vi "FPGAcode4_Test2.vi"() -> ()   [LabVIEW 2015]
uses:
  Limits_In.ctl
  Detector_Cluster.ctl
  <vilib>/Platform/TimedLoop/XDataNode/timing_clust.ctl
  <vilib>/Platform/TimedLoop/XDataNode/nitl_modes.ctl
  <vilib>/Platform/TimedLoop/XDataNode/wakeup.ctl
  Correlations.ctl
  <vilib>/rvi/Emulation/niFpgaGetClockAttributes.vi
  <vilib>/rvi/Emulation/niFpgaSctlEmulationGetInTimedLoop.vi
  <vilib>/rvi/Emulation/niFpgaEmulationReportErrorSimple.vi
  <vilib>/rvi/Emulation/niFpgaProcessEmulError.vi
  <vilib>/rvi/eio/common/nirviEmuTemplateMethod_errors.vi
  <vilib>/rvi/Emulation/niFpgaCriticalErrorInLSC.vi
  <vilib>/eio/EIONode/EIONode.xnode
  <vilib>/Platform/TimedLoop/XDataNode/XDataNode.xnode
  <vilib>/Platform/TimedLoop/XDataNode/XDNodeRunTimeDep.lvlib
panel:
  out "Detectors":T1
  in  "User Trigger?":bool
  in  "User Trigger Distance":fxp<+/-,34,18> format="%.3g"
  out "User Trigger":bool
  in  "Charge Error Factor":fxp<+,32,0>=0.19999999995343387 format="%_2g"
  in  "Threshold Factor":fxp<+/-,32,16>=1.149993896484375 format="%.2g"
  out "DCS 2":bool
  out "DCS 1":bool
  in  "Limits":T2={"High Charge Limit"=4.54747350780585e-13, "Low Charge Limit"=0.0, "High Velocity Limit"=262143.0, "Low Velocity Limit"=0.0, "High Mass Limit"=7.27595761248936e-12, "Low Mass Limit"=0.0, "High Voltage"=2200000.0}
  in  "Calibrate":bool=TRUE
  in  "Armed":bool
  out "Plates":bool
  in  "One Shot":bool
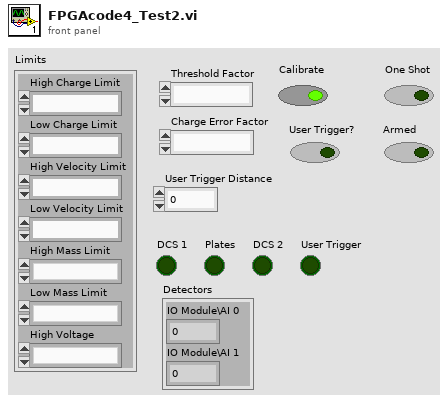
[diagram p1: front panel]
types:
  T1 = cluster{"IO Module\\AI 0":i16, "IO Module\\AI 1":i16}
  T2 = typedef "Limits_In.ctl" = cluster{"High Charge Limit":fxp<+,32,-41>, "Low Charge Limit":fxp<+,32,-41>, "High Velocity Limit":fxp<+,18,18>, "Low Velocity Limit":fxp<+,18,18>, "High Mass Limit":fxp<+/-,33,-36>, "Low Mass Limit":fxp<+/-,33,-36>, "High Voltage":fxp<+,32,22>}
  T3 = typedef "Detector_Cluster.ctl" = cluster{"Det 1":i32, "Det 2":i32}
  T4 = cluster{"Filter 1":T3, "Filter 2":T3, "Filter 3":T3, "Filter 4":T3}
  T5 = cluster{"Distance to PSU":fxp<+/-,32,5>, "Distance to end of PSU":fxp<+/-,32,5>, "Distance to DCS 2":fxp<+/-,32,5>, "Distance to DCS 1":fxp<+/-,32,5>, "Distance to front of LEIL Chamber":fxp<+/-,32,5>}
  T6 = cluster{"Detector Max Speed Count":i32, "Detector Min Speed Count":i32, "Gap Max Speed Count":i32, "Gap Min Speed Count":i32}
  T7 = cluster{"Distance to PSU":fxp<+/-,64,37>, "Distance to end of PSU":fxp<+/-,64,37>, "Distance to DCS 2":fxp<+/-,64,37>, "Distance to DCS 1":fxp<+/-,64,37>, "Distance to front of LEIL Chamber":fxp<+/-,64,37>}
  T8 = cluster{"Filter 1":T3, "Filter 2":T3, "Filter 3":T3, "Filter 4":T3}[]
  T9 = typedef "XDNodeRunTimeDep.lvlib/timing_clust.ctl" = cluster{"Expected End [f-1]":u64, "Actual End [f-1]":u64, "Finished Late? [f-1]":bool, "Expected End [i-1]":u64, "Actual End [i-1]":u64, "Finished Late? [i-1]":bool, "Expected Start [i]":u64, "Actual Start [i]":u64, "Expected Start [f]":u64, "Actual Start [f]":u64, "Source Name":string, "Structure Name":string, "Period":i64, "Deadline":i64, "Offset":i64, "Start":i64, "Priority":i32, "Timeout":i32, "Mode":T10, "Wakeup Reason":T11, "Error":errorcluster, "Source Type":string, "Secondary Source Type":string, "Global End Time":u64, "Global Start Time":u64, "Frame Duration":u64, "Iteration Duration":u64, "Assigned CPU":i32, "I/O Scan Engine Mode":u32}
  T10 = typedef "XDNodeRunTimeDep.lvlib/nitl_modes.ctl" = enum32{"No Change", "Process missed periods, maintain original phase", "Discard missed periods, maintain original phase", "Process missed periods, ignore original phase", "Discard missed periods, ignore original phase"}
  T11 = typedef "XDNodeRunTimeDep.lvlib/wakeup.ctl" = enum32{"Normal", "Aborted", "Asynchronous wakeup", "Timing source error", "Timed loop error", "Timeout"}
  T12 = cluster{"First Detector Count":i32, "Detector Gap Count":i32, "Second Detector Count":i32, "Second Detector Final Count":i32}
  T13 = typedef "Correlations.ctl" = cluster{"First Correlation":i32, "Latest Correlation":i32}
  T14 = cluster{"Distance to PSU":i32, "Distance to end of PSU":i32, "Distance to DCS 2":i32, "Distance to DCS 1":i32, "Distance to front of LEIL Chamber":i32}
  T15 = cluster{"Detectors":cluster{"IO Module\\AI 0":i16, "IO Module\\AI 1":i16}, cluster{"Det 1":i16, "Det 2":i16}, cluster{"Det 1":i16, "Det 2":i16}, cluster{"Det 1":i16, "Det 2":i16}}
  T16 = cluster{cluster{"Det 1":i16, "Det 2":i16}, cluster{"Det 1":i16, "Det 2":i16}, cluster{"Det 1":i16, "Det 2":i16}, cluster{"Det 1":i16, "Det 2":i16}}
  T17 = cluster{"fixed-point type":fxp<+,32,28>, fxp<+/-,64,-6>, fxp<+/-,64,-16>}
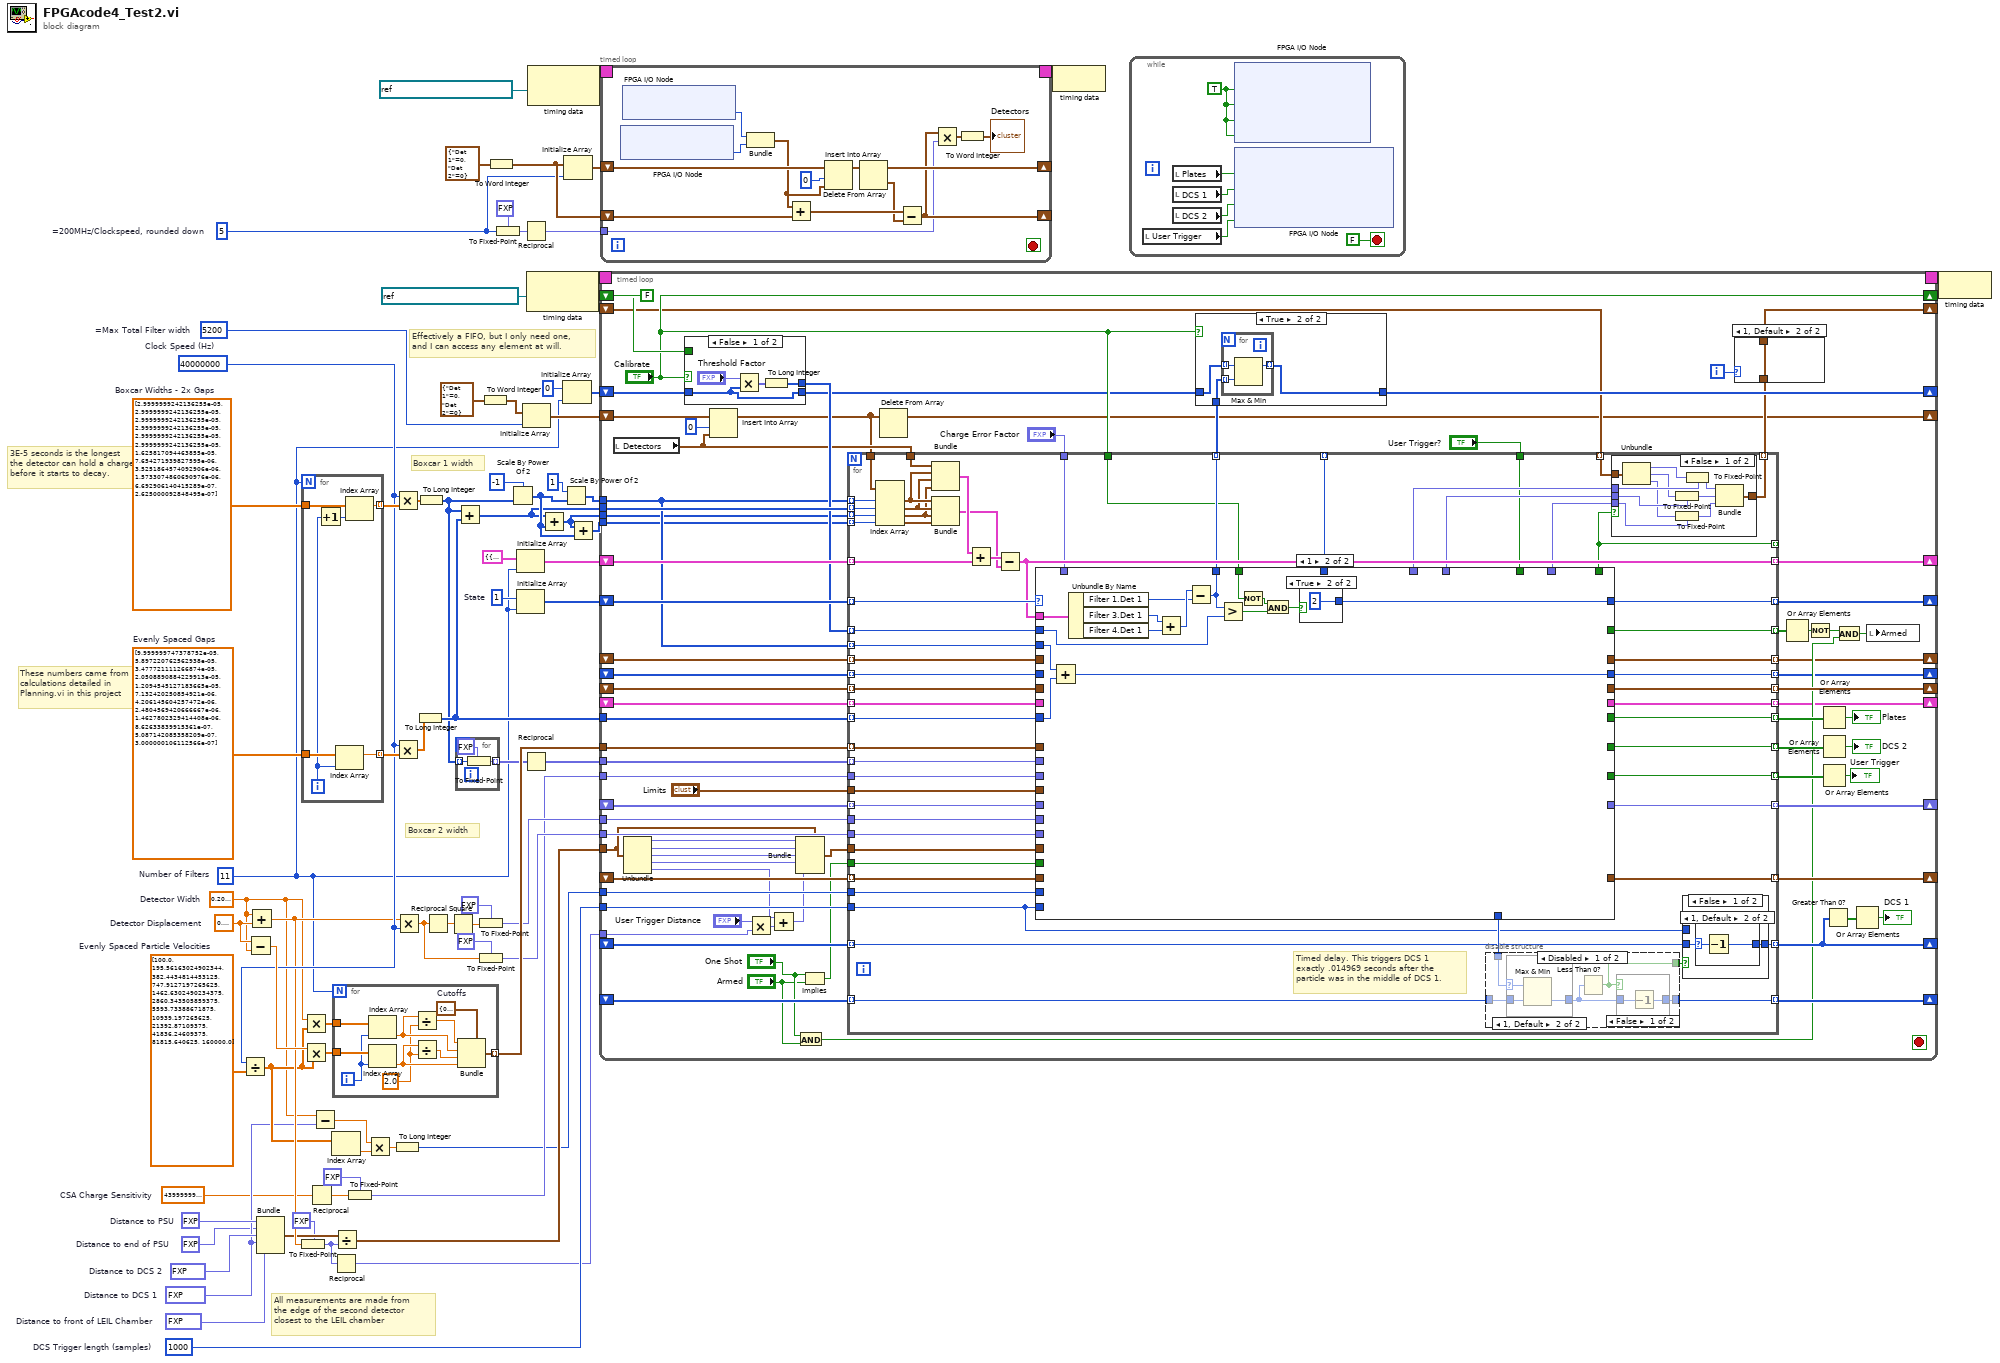
[diagram p0: block diagram]
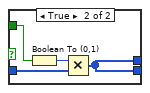
[diagram p3: hidden frame]
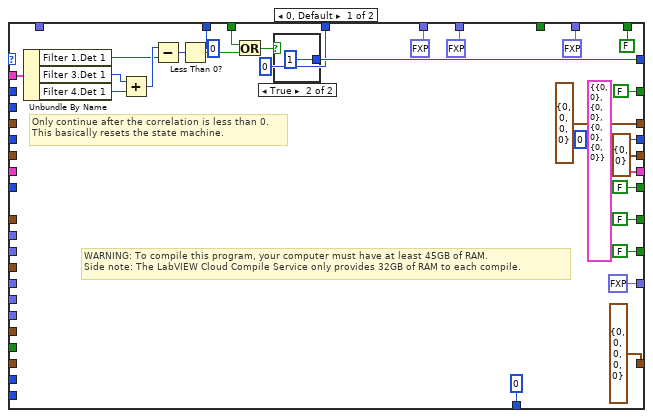
[diagram p5: hidden frame]
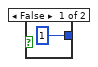
[diagram p7: hidden frame]
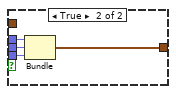
[diagram p8: hidden frame]
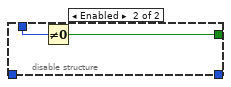
[diagram p13: hidden frame]
diagram:
  w4 = u8 5  # =200MHz/Clockspeed, rounded down
  w11 = 5200  # =Max Total Filter width
  w57 = 40000000  # Clock Speed (Hz)
  w18 = sgl[] [3e-05, 3e-05, 3e-05, 3e-05, 3e-05, 3e-05, 1.6258171e-05, 7.654272e-06, 3.5251865e-06, 1.5733075e-06, 6.692906e-07, 2.625e-07]  # Boxcar Widths - 2x Gaps
  w30 = fxp<+/-,32,5> 4.297679997980595  # Distance to front of LEIL Chamber
  w35 = u16 1000  # DCS Trigger length (samples)
  w40 = fxp<+/-,32,5> -1.3589000031352043  # Distance to DCS 1
  w43 = fxp<+/-,32,5> 2.6162000000476837  # Distance to DCS 2
  w33 = fxp<+/-,32,5> 2.0  # Distance to end of PSU
  w44 = fxp<+/-,32,5> 1.0  # Distance to PSU
  w29 = sgl 4400000000000000.0  # CSA Charge Sensitivity
  w74 = u8 1  # State
  w41 = sgl 0.6  # Detector Displacement
  w69 = sgl[] [0.0001, 5.8972208e-05, 3.477721e-05, 2.050889e-05, 1.2094545e-05, 7.1324203e-06, 4.2061456e-06, 2.480457e-06, 1.4627802e-06, 8.6263384e-07, 5.087142e-07, 3e-07]  # Evenly Spaced Gaps
  w60 = sgl[] [100.0, 195.56163, 382.44348, 747.9127, 1462.6302, 2860.3435, 5593.734, 10939.197, 21392.871, 41836.246, 81815.64, 160000.0]  # Evenly Spaced Particle Velocities
  w36 = sgl 0.21  # Detector Width
  w12 = 11  # Number of Filters
  # "All measurements are made from\nthe edge of the second detector\nclosest to the LEIL chamber"
  # "Effectively a FIFO, but I only need one,\nand I can access any element at will."
  # "Boxcar 2 width"
  # "Boxcar 1 width"
  # "3E-5 seconds is the longest\nthe detector can hold a charge\nbefore it starts to decay."
  # "These numbers came from\ncalculations detailed in\nPlanning.vi in this project"
  n1 = Divide(x=w57, y=w60) -> (x/y=w42:sgl[])
  n2 = Subtract(x=w41, y=w36) -> (x-y=w59:sgl)
  n3 = Add(x=w36, y=w41) -> (x+y=w47:sgl)
  n4 = Bundle("Distance to PSU"=w44, "Distance to end of PSU"=w33, "Distance to DCS 2"=w43, "Distance to DCS 1"=w40, "Distance to front of LEIL Chamber"=w30) -> (w46:T5)  [unwired: 1 in]
  n5 = To Fixed-Point(fixed-point type=fxp<+/-,32,1> 0.0, number=w47) -> (fixed-point=w32:fxp<+/-,32,1>)
  n6 = for {
    N: w12 -> [_]
    tunnel: w69 -> [w84]
    tunnel: [w81] -> w68 mode=indexing
    tunnel: w18 -> [w83]
    tunnel: [w82] -> w67 mode=indexing
    i -> [w80]
    n7 = Increment(x=w80) -> (x+1=w79:i32)
    n8 = Index Array(array=w84, index=w80) -> (element=w81:sgl)
    n9 = Index Array(array=w83, index=w79) -> (element=w82:sgl)
  }
  n10 = Multiply(x=w36, y=w42) -> (x*y=w76:sgl[])
  n11 = Multiply(x=w59, y=w42) -> (x*y=w77:sgl[])
  n12 = Reciprocal(x=w29) -> (1/x=w49:sgl)
  n13 = Subtract(x=w36, y=w40) -> (x-y=w38:sgl)
  n14 = Index Array(array=w42) -> (element=w39:sgl)  [unwired: 1 in]
  n15 = Reciprocal(x=w32) -> (1/x=w31:fxp<+/-,34,33>)
  n16 = for {
    N: w12 -> [_]
    tunnel: w77 -> [w94]
    tunnel: w76 -> [w93]
    tunnel: [w92] -> w71 mode=indexing
    i -> [w91]
    w85 = sgl 2.0 ("y")
    w90 = T6 {"Detector Max Speed Count"=0, "Detector Min Speed Count"=0, "Gap Max Speed Count"=0, "Gap Min Speed Count"=0}  # Cutoffs
    n17 = Index Array(array=w93, index=w91) -> (element=w89:sgl)
    n18 = Index Array(array=w94, index=w91) -> (element=w86:sgl)
    n19 = Divide(x=w89, y=w85) -> (x/y=w88:sgl)
    n20 = Divide(x=w86, y=w85) -> (x/y=w87:sgl)
    n21 = Bundle(cluster=w90, "Detector Max Speed Count"=w88, "Detector Min Speed Count"=w89, "Gap Max Speed Count"=w87, "Gap Min Speed Count"=w86) -> (w92:T6)
  }
  n22 = Divide(x=w46, y=w32) -> (x/y=w45:T7)
  n23 = To Fixed-Point(fixed-point type=fxp<+,32,-49> 0.0, number=w49) -> (fixed-point=w48:fxp<+,32,-49>)
  n24 = Multiply(x=w38, y=w39) -> (x*y=w37:sgl)
  n25 = To Long Integer(number=w37) -> (32bit integer=w34:i32)
  n26 = Multiply(x=w57, y=w67) -> (x*y=w70:sgl[])
  n27 = Multiply(x=w57, y=w68) -> (x*y=w75:sgl[])
  n28 = Multiply(x=w47, y=w57) -> (x*y=w52:sgl)
  n29 = To Long Integer(number=w75) -> (32bit integer=w66:i32[])
  n30 = To Long Integer(number=w70) -> (32bit integer=w23:i32[])
  n31 = Reciprocal(x=w52) -> (1/x=w56:sgl)
  n32 = Square(x=w56) -> (x^2=w55:sgl)
  n33 = Add(x=w23, y=w66) -> (x+y=w19:i32[])
  n34 = for {
    tunnel: w23 -> [w97] mode=indexing
    tunnel: [w96] -> w62 mode=indexing
    n35 = To Fixed-Point(fixed-point type=fxp<+/-,32,32> 0.0, number=w97) -> (fixed-point=w96:fxp<+/-,32,32>)
  }
  n36 = To Fixed-Point(fixed-point type=fxp<+/-,32,-42> 0.0, number=w55) -> (fixed-point=w58:fxp<+/-,32,-42>)
  n37 = To Fixed-Point(fixed-point type=fxp<+,32,28> 0.0, number=w52) -> (fixed-point=w50:fxp<+,32,28>)
  n38 = To Word Integer(number=T3 {"Det 1"=0, "Det 2"=0} ("Detectors")) -> (16bit integer=w65:cluster{"Det 1":i16, "Det 2":i16})
  n39 = To Word Integer(number=T3 {"Det 1"=0, "Det 2"=0} ("Detectors")) -> (16bit integer=w5:cluster{"Det 1":i16, "Det 2":i16})
  n40 = To Fixed-Point(fixed-point type=fxp<+,4,4> 0.0, number=w4) -> (fixed-point=w3:fxp<+,4,4>)
  n41 = Scale By Power Of 2(n=i16 -1, x=w23) -> (x*2^n=w21:i32[])
  n42 = Initialize Array(T4 {"Filter 1"={"Det 1"=0, "Det 2"=0}, "Filter 2"={"Det 1"=0, "Det 2"=0}, "Filter 3"={"Det 1"=0, "Det 2"=0}, "Filter 4"={"Det 1"=0, "Det 2"=0}} ("cluster"), w12) -> (w72:T8)
  n43 = Initialize Array(w74, w12) -> (w73:u8[])
  n44 = Reciprocal(x=w3) -> (1/x=w2:fxp<+,5,1>)
  n45 = Initialize Array(w65, w11) -> (w78:cluster{"Det 1":i16, "Det 2":i16}[])
  n46 = Reciprocal(x=w62) -> (1/x=w61:fxp<+/-,34,2>[])
  n47 = node-c288(refnum<k21> "40 MHz Onboard Clock" ("Source Name")) -> (w17:T9)
  n48 = node-c288(refnum<k21> "IO Module\\Data Clock" ("Source Name")) -> (w10:T9)
  n49 = Add(x=w19, y=w21) -> (x+y=w22:i32[])
  n50 = Scale By Power Of 2(n=i16 1, x=w21) -> (x*2^n=w26:i32[])
  n51 = Initialize Array(0 ("Thresholds in"), w12) -> (w13:i32[])
  n52 = Initialize Array(w5, w4) -> (w7:cluster{"Det 1":i16, "Det 2":i16}[])
  n53 = Add(x=w22, y=w21) -> (x+y=w20:i32[])
  n54 = timed-loop {
    shift-right: [w98] -> _
    shift-left: w78 -> [w175]
    shift-right: [w107] -> _
    shift-left: w72 -> [w172]
    shift-right: [w101] -> _
    shift-left: w73 -> [w174]
    shift-right: [w108] -> _
    shift-left: _ -> [w173]
    tunnel: w71 -> [w171]
    shift-right: [w170] -> _
    shift-left: _ -> [w169]
    tunnel: w26 -> [w106]
    tunnel: w19 -> [w168]
    tunnel: w66 -> [w167]
    tunnel: w61 -> [w166]
    shift-right: [w165] -> _
    shift-left: _ -> [w164]
    tunnel: w58 -> [w163]
    tunnel: w48 -> [w162]
    tunnel: w50 -> [w161]
    tunnel: w45 -> [w148]
    shift-right: [w160] -> _
    shift-left: _ -> [w159]
    shift-right: [w158] -> _
    shift-left: w13 -> [w157]
    shift-right: ["Calibrate"] -> _
    shift-left: FALSE ("Calibrate") -> [w156]
    tunnel: w35 -> [w155]
    tunnel: w34 -> [w154]
    shift-right: [w152] -> _
    shift-left: _ -> [w153]
    shift-right: [w151] -> _
    shift-left: _ -> [w150]
    tunnel: w31 -> [w149]
    shift-right: [w117] -> _
    shift-left: _ -> [w116]
    shift-right: [w110] -> _
    shift-left: _ -> [w112]
    shift-right: [w105] -> _
    shift-left: _ -> [w104]
    tunnel: w20 -> [w103]
    tunnel: w22 -> [w102]
    timing: w17 -> [_]
    timing-out: [_] -> w16
    i -> [w111]
    stop <- _ stop-if-true
    n55 = local read "Detectors"() -> (w100:T1)
    n56 = Unbundle(w148) -> ("Distance to PSU"=w139:fxp<+/-,64,37>, "Distance to end of PSU"=w138:fxp<+/-,64,37>, "Distance to DCS 2"=w137:fxp<+/-,64,37>, "Distance to DCS 1"=w134:fxp<+/-,64,37>, "Distance to front of LEIL Chamber"=w133:fxp<+/-,64,37>)
    n57 = case shown="False" "Calibrate" {
      tunnel: w157 -> [w178 w184]
      tunnel: [w178 w181] -> w113
      tunnel: w156 -> [_ w183]
      tunnel: [w177 w181] -> w114
      frame False {
        n58 = Multiply(x="Threshold Factor", y=w178) -> (x*y=w179:fxp<+/-,64,48>[])
        n59 = To Long Integer(number=w179) -> (32bit integer=w177:i32[])
      }
      frame True {
        n60 = Boolean To (0,1)(Boolean=w183) -> (0, 1=w182:i16)
        n61 = Multiply(x=w182, y=w184) -> (x*y=w181:i32[])
      }
    }
    n62 = Insert Into Array(array=w175, index=0, new element=w100) -> (w99:cluster{"Det 1":i16, "Det 2":i16}[])
    n63 = Multiply(x="User Trigger Distance", y=w149) -> (x*y=w135:fxp<+/-,64,49>)
    n64 = Add(x=w133, y=w135) -> (x+y=w132:fxp<+/-,64,50>)
    n65 = Bundle(cluster=w148, "Distance to PSU"=w139, "Distance to end of PSU"=w138, "Distance to DCS 2"=w137, "Distance to DCS 1"=w134, "Distance to front of LEIL Chamber"=w132) -> (w136:T7)
    n66 = And(x="One Shot", y="Armed") -> (x .and. y?=w123:bool)
    n67 = Implies(1:"Armed", 2:"One Shot") -> (0:w143:bool)
    n68 = for {
      tunnel: w99 -> [w254]
      tunnel: [w240] -> w107 mode=indexing
      tunnel: w174 -> [w253] mode=indexing
      tunnel: [w252] -> w101 mode=indexing
      tunnel: w114 -> [w195] mode=indexing
      tunnel: [w251] -> w108 mode=indexing
      tunnel: w173 -> [w250] mode=indexing
      tunnel: w172 -> [w244] mode=indexing
      tunnel: w100 -> [w249]
      tunnel: w171 -> [w239] mode=indexing
      tunnel: [w238] -> w170 mode=indexing
      tunnel: w169 -> [w237] mode=indexing
      tunnel: w106 -> [w236] mode=indexing
      tunnel: w168 -> [w193] mode=indexing
      tunnel: w102 -> [w235] mode=indexing
      tunnel: w103 -> [w234] mode=indexing
      tunnel: w106 -> [w199] mode=indexing
      tunnel: w167 -> [w198] mode=indexing
      tunnel: "Charge Error Factor" -> [w233]
      tunnel: [w232] -> _ mode=indexing
      tunnel: w166 -> [w231] mode=indexing
      tunnel: "Limits" -> [w230]
      tunnel: [w229] -> w165 mode=indexing
      tunnel: w164 -> [w228] mode=indexing
      tunnel: w163 -> [w227]
      tunnel: w162 -> [w226]
      tunnel: w161 -> [w225]
      tunnel: w136 -> [w224]
      tunnel: [w223] -> w160 mode=indexing
      tunnel: w159 -> [w222] mode=indexing
      tunnel: [w221] -> w144 mode=indexing
      tunnel: w143 -> [w220]
      tunnel: w155 -> [w217]
      tunnel: w154 -> [w219]
      tunnel: [w216] -> w152 mode=indexing
      tunnel: w153 -> [w215] mode=indexing
      tunnel: [w213] -> w151 mode=indexing
      tunnel: w150 -> [w212] mode=indexing
      tunnel: [w211] -> w131 mode=indexing
      tunnel: [w210] -> w130 mode=indexing
      tunnel: [w209] -> w129 mode=indexing
      tunnel: [w208] -> w126 mode=indexing
      tunnel: "User Trigger?" -> [w204]
      tunnel: w116 -> [w203] mode=indexing
      tunnel: [w202] -> w117 mode=indexing
      tunnel: "Calibrate" -> [w201]
      tunnel: [w197] -> w109 mode=indexing
      tunnel: w112 -> [w200] mode=indexing
      tunnel: [w196] -> _ mode=indexing
      tunnel: [w194] -> w105 mode=indexing
      tunnel: w104 -> [w192] mode=indexing
      # "Timed delay. This triggers DCS 1\nexactly .014969 seconds after the\nparticle was in the middle of DCS 1."
      n69 = Index Array(array=w254, index #1=w236, index #2=w193, index #3=w235, index #4=w234) -> (element #1=w247:cluster{"Det 1":i16, "Det 2":i16}, element #2=w246:cluster{"Det 1":i16, "Det 2":i16}, element #3=w245:cluster{"Det 1":i16, "Det 2":i16}, element #4=w248:cluster{"Det 1":i16, "Det 2":i16})
      n70 = Bundle("Detectors"=w249, w247, w246, w245) -> (w243:T15)  [unwired: 1 in]
      n71 = Bundle(w247, w246, w245, w248) -> (w241:T16)  [unwired: 1 in]
      n72 = Add(x=w243, y=w244) -> (x+y=w242:T4)
      n73 = Subtract(x=w242, y=w241) -> (x-y=w240:T4)
      n74 = case shown="1" w253 {
        tunnel: w195 -> [_ w297]
        tunnel: [w280 w295] -> w252
        tunnel: w199 -> [_ w285]
        tunnel: [T12 {"First Detector Count"=0, "Detector Gap Count"=0, "Second Detector Count"=0, "Second Detector Final Count"=0} ("Cutoffs") _] -> w251
        tunnel: w250 -> [_ _]
        tunnel: w192 -> [_ _]
        tunnel: w240 -> [w275 w290]
        tunnel: w239 -> [_ _]
        tunnel: w237 -> [_ _]
        tunnel: w198 -> [_ w284]
        tunnel: w233 -> [_ _]
        tunnel: [u8 0 ("Det 3") _] -> w232
        tunnel: w231 -> [_ _]
        tunnel: w230 -> [_ _]
        tunnel: [fxp<+/-,64,-16> 0.0 _] -> w229
        tunnel: w228 -> [_ _]
        tunnel: w227 -> [_ _]
        tunnel: w226 -> [_ _]
        tunnel: w225 -> [_ _]
        tunnel: w224 -> [_ _]
        tunnel: [T14 {"Distance to PSU"=0, "Distance to end of PSU"=0, "Distance to DCS 2"=0, "Distance to DCS 1"=0, "Distance to front of LEIL Chamber"=0} _] -> w223
        tunnel: w222 -> [_ _]
        tunnel: [0 w289] -> w221
        tunnel: w220 -> [_ _]
        tunnel: w219 -> [_ _]
        tunnel: w217 -> [_ _]
        tunnel: [0 _] -> w218
        tunnel: [FALSE _] -> w211
        tunnel: [FALSE _] -> w210
        tunnel: [FALSE _] -> w209
        tunnel: [FALSE _] -> w208
        tunnel: [fxp<+,32,28> 0.0 ("fixed-point type") _] -> w205
        tunnel: [fxp<+/-,64,-16> 0.0 _] -> w207
        tunnel: [fxp<+/-,64,-6> 0.0 _] -> w206
        tunnel: w204 -> [_ _]
        tunnel: [T4 {"Filter 1"={"Det 1"=0, "Det 2"=0}, "Filter 2"={"Det 1"=0, "Det 2"=0}, "Filter 3"={"Det 1"=0, "Det 2"=0}, "Filter 4"={"Det 1"=0, "Det 2"=0}} _] -> w202
        tunnel: w203 -> [_ _]
        tunnel: [FALSE ("result") _] -> w196
        tunnel: w201 -> [w272 w286]
        tunnel: [0 w283] -> w194
        tunnel: [T13 {"First Correlation"=0, "Latest Correlation"=0} ("cluster") _] -> w238
        frame 0, Default {
          # "WARNING: To compile this program, your computer must have at least 45GB of RAM.\nSide note: The LabVIEW Cloud Compile Service only provides 32GB of RAM to each compile."
          # "Only continue after the correlation is less than 0.\nThis basically resets the state machine."
          n75 = Unbundle By Name(w275) -> ("Filter 1.Det 1"=w276:i32, "Filter 3.Det 1"=w277:i32, "Filter 4.Det 1"=w278:i32)
          n76 = Add(x=w277, y=w278) -> (x+y=w279:i32)
          n77 = Subtract(x=w279, y=w276) -> (x-y=w274:i32)
          n78 = Less Than 0?(x=w274) -> (x < 0?=w281:bool)
          n79 = Or(x=w272, y=w281) -> (x .or. y?=w273:bool)
          n80 = case shown="True" w273 {
            tunnel: [_ u8 1 ("Det 3")] -> w280
            frame False {
            }
            frame True {
            }
          }
        }
        frame 1 {
          n81 = Add(x=w285, y=w284) -> (x+y=w283:i32)
          n82 = Unbundle By Name(w290) -> ("Filter 1.Det 1"=w291:i32, "Filter 3.Det 1"=w292:i32, "Filter 4.Det 1"=w293:i32)
          n83 = Add(x=w292, y=w293) -> (x+y=w294:i32)
          n84 = Subtract(x=w294, y=w291) -> (x-y=w289:i32)
          n85 = Greater?(x=w289, y=w297) -> (0:w296:bool)
          n86 = Not(x=w286) -> (.not. x?=w287:bool)
          n87 = And(x=w287, y=w296) -> (x .and. y?=w288:bool)
          n88 = case shown="True" w288 {
            tunnel: [u8 1 ("Det 3") u8 2 ("Det 3")] -> w295
            frame False {
            }
            frame True {
            }
          }
        }
      }
      n89 = disable-structure shown="Disabled" {
        disable-tunnel: w218 -> [w325 w333]
        disable-tunnel: [w321 w332] -> w214
        disable-tunnel: [w323 _] -> w213
        disable-tunnel: w212 -> [w324 _]
        frame Disabled {
          n90 = case shown="1, Default" w325 {
            selector: w325 -> [_ w331]
            tunnel: [w328 w329] -> w322
            tunnel: w324 -> [w328 w330]
            frame 0 {
            }
            frame 1, Default {
              n91 = Max & Min(x=w331, y=w330) -> (min(x,y)=w329:i32)  [unwired: 1 out]
            }
          }
          n92 = Less Than 0?(x=w322) -> (x < 0?=w321:bool)
          n93 = case shown="False" w321 {
            tunnel: w322 -> [w327 _]
            tunnel: [w326 _] -> w323
            frame False {
              n94 = Decrement(x=w327) -> (x-1=w326:i32)
            }
            frame True {
            }
          }
        }
        frame Enabled {
          n95 = Not Equal To 0?(x=w333) -> (x != 0?=w332:bool)
        }
      }
      n96 = case shown="False" w196 {
        tunnel: w207 -> [w305 w312]
        tunnel: w206 -> [w306 w313]
        tunnel: w205 -> [w308 w314]
        tunnel: [w303 w311] -> w197
        tunnel: w200 -> [w310 _]
        frame False {
          n97 = Unbundle(w310) -> ("fixed-point type"=w309:fxp<+,32,28>, w307:fxp<+/-,64,-6>, w304:fxp<+/-,64,-16>)
          n98 = To Fixed-Point(fixed-point type=w306, number=w307) -> (fixed-point=w301:fxp<+/-,64,-6>)
          n99 = To Fixed-Point(fixed-point type=w305, number=w304) -> (fixed-point=w300:fxp<+/-,64,-16>)
          n100 = To Fixed-Point(fixed-point type=w308, number=w309) -> (fixed-point=w302:fxp<+,32,28>)
          n101 = Bundle("fixed-point type"=w302, w301, w300) -> (w303:T17)  [unwired: 1 in]
        }
        frame True {
          n102 = Bundle("fixed-point type"=w314, w313, w312) -> (w311:T17)  [unwired: 1 in]
        }
      }
      n103 = case shown="False" w214 {
        tunnel: w217 -> [_ w320]
        tunnel: [w315 w320] -> w216
        tunnel: w215 -> [w316 _]
        frame False {
          n104 = case shown="1, Default" w316 {
            selector: w316 -> [w317 w319]
            tunnel: [w317 w318] -> w315
            frame 0 {
            }
            frame 1, Default {
              n105 = Decrement(x=w319) -> (x-1=w318:u16)
            }
          }
        }
        frame True {
        }
      }
    }
    n106 = Delete From Array(array=w99) -> (array with subset deleted=w98:cluster{"Det 1":i16, "Det 2":i16}[])  [unwired: 2 in, 1 out]
    n107 = case shown="True" "Calibrate" {
      tunnel: w113 -> [w185 w188]
      tunnel: [w185 w186] -> w158
      tunnel: w144 -> [_ w187]
      frame False {
      }
      frame True {
        n108 = for {
          tunnel: w187 -> [w191] mode=indexing
          tunnel: w188 -> [w190] mode=indexing
          tunnel: [w189] -> w186 mode=indexing
          n109 = Max & Min(x=w190, y=w191) -> (max(x,y)=w189:i32)  [unwired: 1 out]
        }
      }
    }
    n110 = case shown="1, Default" w111 {
      tunnel: [_ w176] -> w110
      tunnel: w109 -> [_ w176]
      frame 0 {
      }
      frame 1, Default {
      }
    }
    n111 = Or Array Elements(Boolean array=w126) -> (logical OR=w120:bool)
    n112 = Not(x=w120) -> (.not. x?=w125:bool)
    n113 = Or Array Elements(Boolean array=w131) -> (logical OR=→"Plates":bool)
    n114 = Or Array Elements(Boolean array=w130) -> (logical OR=→"DCS 2":bool)
    n115 = Or Array Elements(Boolean array=w129) -> (logical OR=→"User Trigger":bool)
    n116 = Greater Than 0?(x=w152) -> (x > 0?=w141:bool[])
    n117 = And(x=w125, y=w123) -> (x .and. y?=w124:bool)
    n118 = Or Array Elements(Boolean array=w141) -> (logical OR=→"DCS 1":bool)
    n119 = local write "Armed"(w124) -> ()
  }
  n120 = timed-loop {
    timing: w10 -> [_]
    timing-out: [_] -> w9
    shift-right: [w344] -> _
    shift-left: w7 -> [w345]
    shift-right: [w339] -> _
    shift-left: w5 -> [w343]
    tunnel: w2 -> [w338]
    stop <- _ stop-if-true
    n121 = xnode "FPGA I/O Node"() -> ("IO Module\\AI 1"=w348:i16)  [unwired: 1 in, 1 out]
    n122 = xnode "FPGA I/O Node"() -> ("IO Module\\AI 0"=w349:i16)  [unwired: 1 in, 1 out]
    n123 = Bundle("IO Module\\AI 0"=w349, "IO Module\\AI 1"=w348) -> (w340:T1)  [unwired: 1 in]
    n124 = Add(x=w340, y=w343) -> (x+y=w342:cluster{i16, i16})
    n125 = Insert Into Array(array=w345, index=0, new element=w340) -> (w346:cluster{"Det 1":i16, "Det 2":i16}[])
    n126 = Delete From Array(array=w346) -> (deleted portion=w341:cluster{"Det 1":i16, "Det 2":i16}, array with subset deleted=w344:cluster{"Det 1":i16, "Det 2":i16}[])  [unwired: 2 in]
    n127 = Subtract(x=w342, y=w341) -> (x-y=w339:cluster{i16, i16})
    n128 = Multiply(x=w339, y=w338) -> (x*y=w337:cluster{fxp<+/-,20,16>, fxp<+/-,20,16>})
    n129 = To Word Integer(number=w337) -> (16bit integer=→"Detectors":cluster{i16, i16})
  }
  n130 = node-c288(w9) -> ()
  n131 = while {
    stop <- FALSE stop-if-true
    w355 = TRUE ("IO Module\\PFI Enable")
    n132 = local read "User Trigger"() -> (w353:bool)
    n133 = local read "Plates"() -> (w356:bool)
    n134 = local read "DCS 1"() -> (w354:bool)
    n135 = local read "DCS 2"() -> (w352:bool)
    n136 = xnode "FPGA I/O Node"("IO Module\\PFI 0 WE"=w355, "IO Module\\PFI 1 WE"=w355, "IO Module\\PFI 2 WE"=w355, "IO Module\\PFI 3 WE"=w355) -> ()  [unwired: 4 in, 4 out]
    n137 = xnode "FPGA I/O Node"("IO Module\\PFI 0 Wr Data"=w356, "IO Module\\PFI 1 Wr Data"=w354, "IO Module\\PFI 2 Wr Data"=w352, "IO Module\\PFI 3 Wr Data"=w353) -> ()  [unwired: 4 in, 4 out]
  }
  n138 = node-c288(w16) -> ()
